vi "Drive for Distance.vi"(6 "Synchronication":enum16{"Start", "Wait"}(ring)=enum."Wait", 7 "Description":string, 8 "Command Info In":T1, 11 "Distance (in.)":dbl) -> (0 "Command Info Out":T1)   [LabVIEW 2019]
doc: "This VI notifies the subsystem to perform this command for the given duration, then go back to the default state. Synchronization determines whether this VI Starts the operation and returns immediately, or waits for the operation to complete. The first option is commonly used for TeleOp, and the second for Autonomous sequencing."
uses:
  <vilib>/Rock Robotics/WPI/Framework/Command Status Info.ctl
  <vilib>/Rock Robotics/WPI/Framework/Completion Status.ctl
  <vilib>/Rock Robotics/WPI/Framework/Completion Notifier.ctl
  Implementation/Drive Setpoints.ctl
  Implementation/Drive Operations.ctl
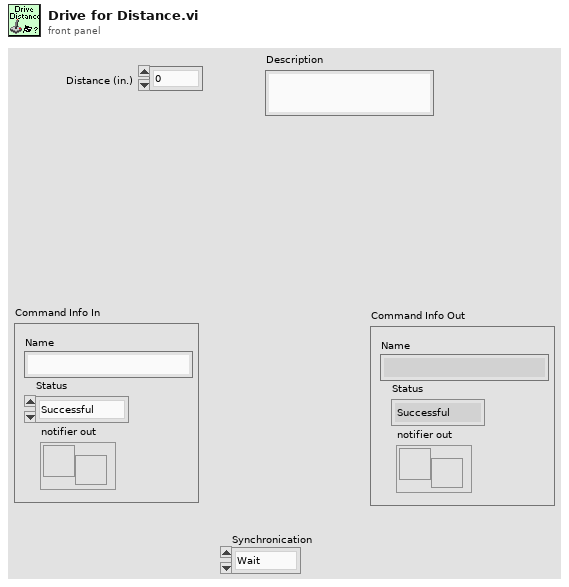
[diagram p1: front panel]
types:
  T1 = typedef "Command Status Info.ctl" = cluster{"Name":string, "Status":T2, "notifier out":T3}
  T2 = typedef "Completion Status.ctl" = enum16{"Successful", "Aborted", "Incomplete"}
  T3 = typedef "Completion Notifier.ctl" = refnum<notifier>
  T4 = typedef "Drive Setpoints.ctl" = cluster{"Operation":T5, "Left Setpoint":dbl, "Right Setpoint":dbl, "Duration":dbl, "Angle Setpoint":dbl, "Distance Setpoint":dbl}
  T5 = typedef "Drive Operations.ctl" = enum16{"Reserve", "Read Current", "Arcade Drive Immediate", "Arcade Drive Straight Immediate", "Drive for Time", "Turn By Angle", "Drive for Distance"}
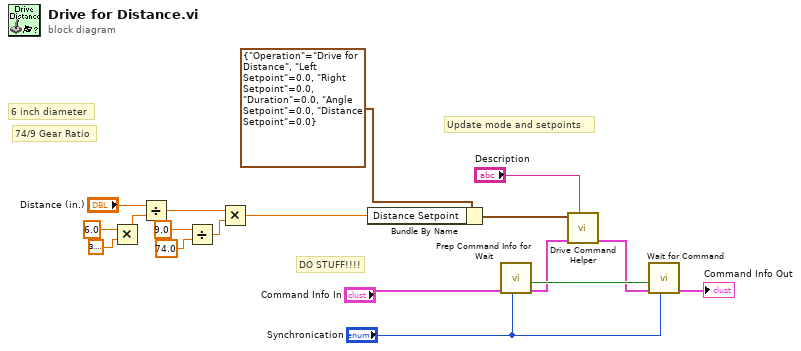
[diagram p0: block diagram]
diagram:
  # "74/9 Gear Ratio"
  # "6 inch diameter"
  # "DO STUFF!!!!"
  # "Update mode and setpoints"
  n1 = Multiply(x=6.0, y=3.141592653589793) -> (x*y=w4:dbl)
  n2 = Divide(x="Distance (in.)", y=w4) -> (x/y=w2:dbl)
  n3 = Divide(x=9.0, y=74.0) -> (x/y=w9:dbl)
  n4 = Multiply(x=w2, y=w9) -> (x*y=w1:dbl)
  n5 = Bundle By Name(cluster=T4 {"Operation"=enum."Drive for Distance", "Left Setpoint"=0.0, "Right Setpoint"=0.0, "Duration"=0.0, "Angle Setpoint"=0.0, "Distance Setpoint"=0.0} ("SubSystem Data"), "Distance Setpoint"=w1) -> (w10:T4)
  n6 = call <vilib>:"Prep Command Info for Wait.vi"("Synchronication"="Synchronication", "Command Info"="Command Info In") -> ("Command Info"=w16:T1, "Allocated"=w17:bool)  [unwired: 8 in]
  n7 = call "Drive Command Helper.vi"("Description"="Description", "Command Info In"=w16, "SubSystem Data"=w10) -> ("Command Info Out"=w13:T1)  [unwired: 6 in, 2 out]
  n8 = call <vilib>:"Wait for Command.vi"("Synchronication"="Synchronication", "Command Info in"=w13, "Allocated"=w17) -> ("Command Info out"=→"Command Info Out":T1)  [unwired: 8 in]
